vi "Result View.vi"(8 "error in (no error)":errorcluster, 11 "Coverage Report in":refnum<class "Coverage Report.lvclass">) -> (0 "error out":errorcluster, 3 "Coverage Report out":refnum<class "Coverage Report.lvclass">)   [LabVIEW 2020, in "Coverage Report.lvclass"]
uses:
  Coverage Report.lvclass
  Coverage Report.lvclass/Coverage Report.ctl
panel:
  in  "VI tree":string[](tree)
  out "Coverage Report Out":refnum<class "Coverage Report.lvclass">
  out "error out 2":errorcluster
  in  "Cancel":bool
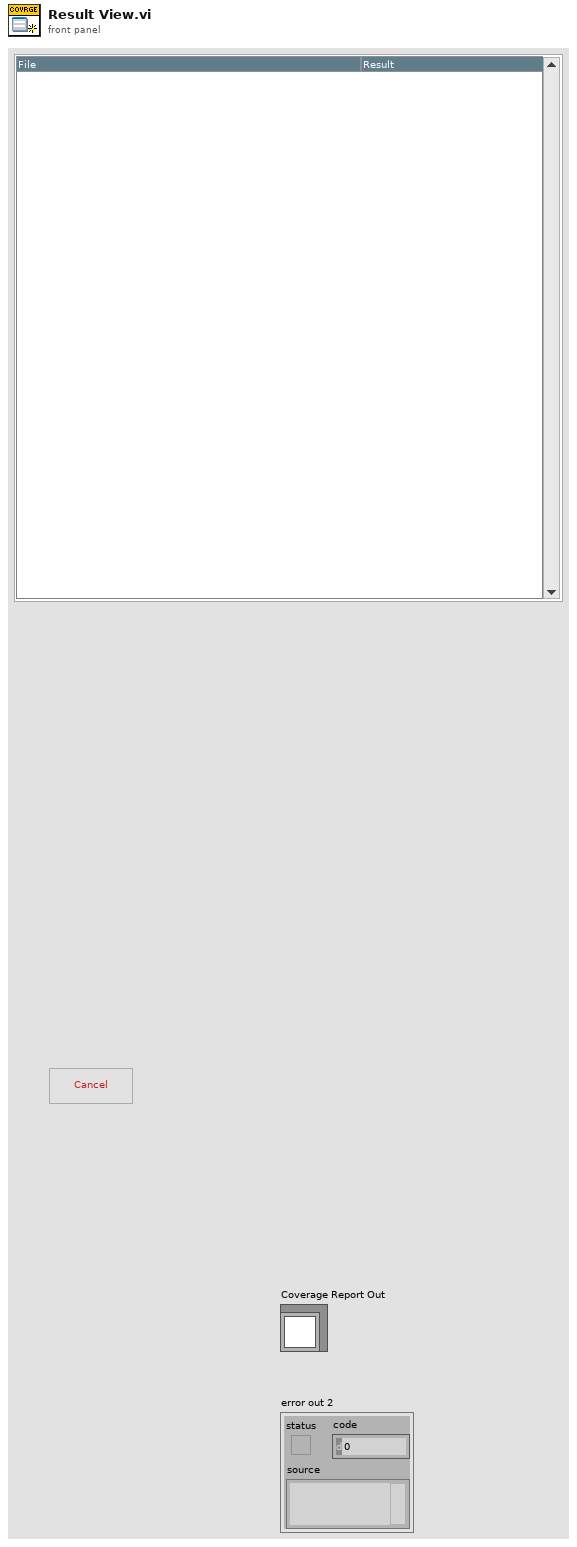
[diagram p1: front panel]
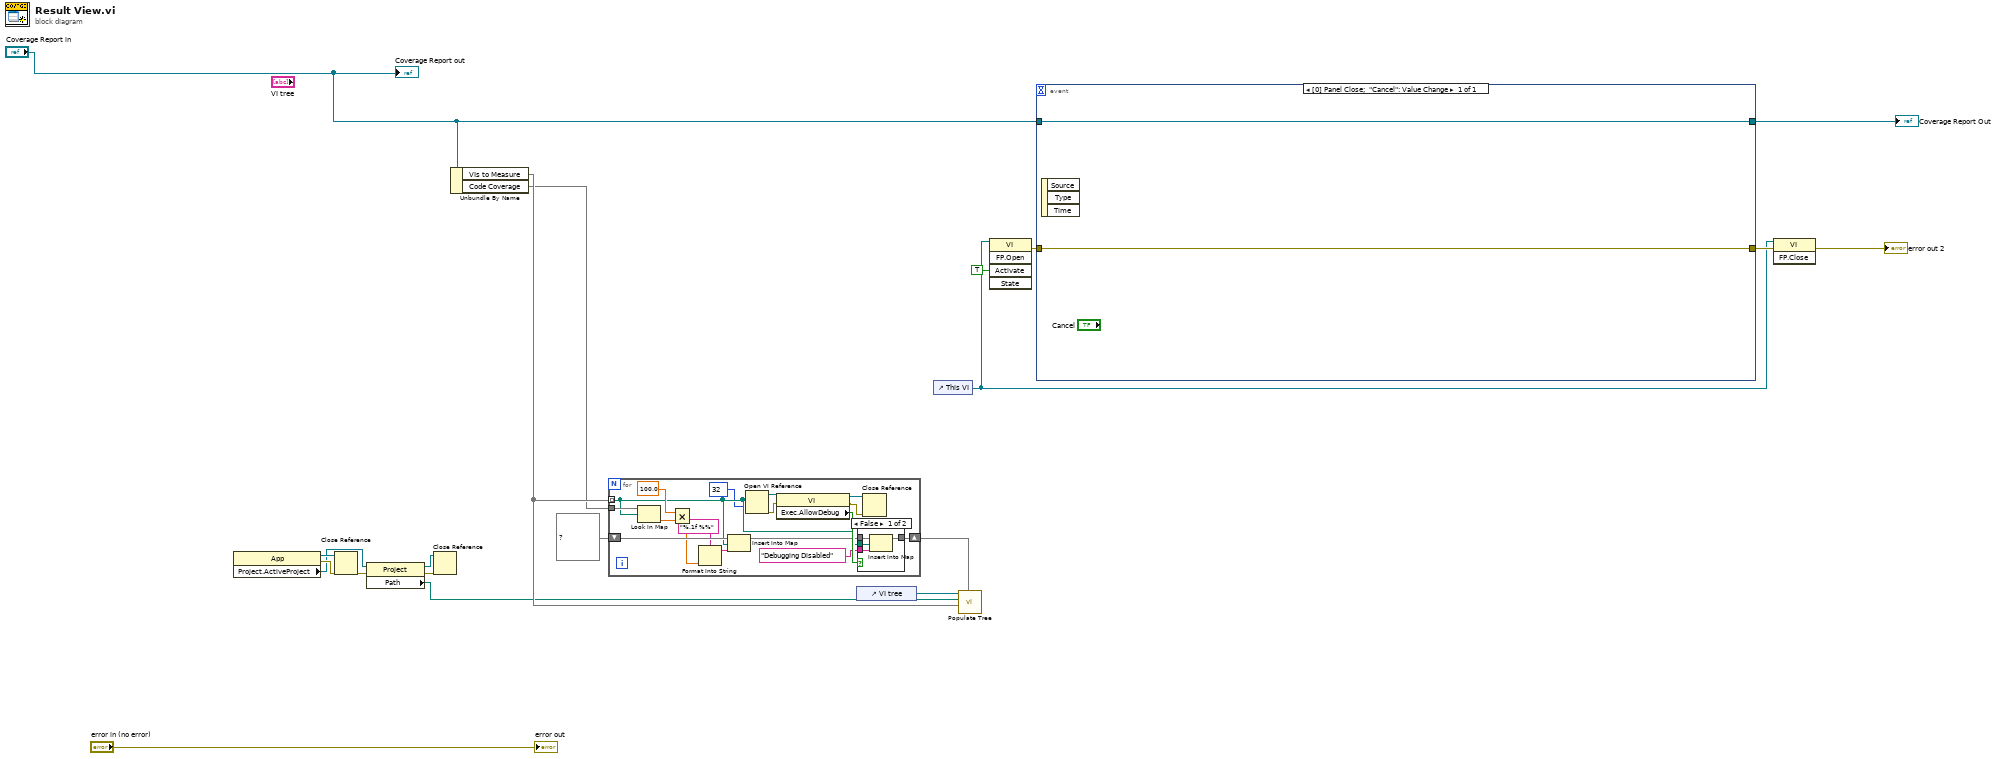
[diagram p0: block diagram]
diagram:
  n1 = property class="App"() -> (reference out=w3:refnum<vi>, error out=w6:errorcluster, "Project.ActiveProject"=w2:refnum<vi>)  [unwired: 2 in]
  n2 = Close Reference(reference=w3, error in (no error)=w6) -> (error out=w7:errorcluster)
  n3 = property class="Project"(reference=w2, error in=w7) -> (reference out=w4:refnum<vi>, error out=w5:errorcluster, "Path"=w1:path)
  n4 = Close Reference(reference=w4, error in (no error)=w5) -> ()  [unwired: 1 out]
  n5 = Unbundle By Name("Coverage Report in") -> ("VIs to Measure"=w9:set{path}, "Code Coverage"=w8:map{path, dbl})
  n6 = for {
    tunnel: w9 -> [w25] mode=indexing
    shift-right: [w32] -> w15
    shift-left: map{path, string} {} ("Results") -> [w36]
    tunnel: w8 -> [w30]
    n7 = Look In Map(map=w30, key=w25) -> (value=w28:dbl)  [unwired: 1 in, 1 out]
    n8 = Multiply(x=100.0, y=w28) -> (x*y=w23:dbl)
    n9 = Format Into String(format string="%.1f %%", w23) -> (resulting string=w26:string)  [unwired: 2 in, 1 out]
    n10 = Insert Into Map(map in=w36, key=w25, value=w26) -> (map out=w29:map{path, string})  [unwired: 2 out]
    n11 = Open VI Reference(vi path=w25, options=32) -> (vi reference=w37:refnum<vi>, error out=w34:errorcluster)  [unwired: 4 in]
    n12 = property class="VI"(reference=w37, error in=w34) -> (reference out=w35:refnum<vi>, error out=w21:errorcluster, "Exec.AllowDebug"=w33:bool)
    n13 = case shown="False" w33 {
      tunnel: w29 -> [w41 w42]
      tunnel: [w40 w42] -> w32
      tunnel: w25 -> [w39 _]
      tunnel: "Debugging Disabled" ("value") -> [w38 _]
      frame False {
        n14 = Insert Into Map(map in=w41, key=w39, value=w38) -> (map out=w40:map{path, string})  [unwired: 2 out]
      }
      frame True {
      }
    }
    n15 = Close Reference(reference=w35, error in (no error)=w21) -> ()  [unwired: 1 out]
  }
  n16 = control-ref of="VI tree"() -> (w17:refnum<vi>)
  n17 = control-ref of="This VI"() -> (w10:refnum<vi>)
  n18 = call "Populate Tree.vi"("Results"=w15, "VIs"=w9, "Project Path"=w1, "TreeControl in"=w17) -> ()  [unwired: 7 in, 1 out]
  n19 = invoke class="VI" method="FP.Open"(reference=w10, "Activate"=TRUE ("Activate?")) -> (error out=w12:errorcluster)  [unwired: 3 in, 4 out]
  n20 = event shown="[0] Panel Close;  \"Cancel\": Value Change" {
    selector: _ -> [_]
    dyn-events: _ -> [_]
    timeout: _ -> [_]
    tunnel: w12 -> [w44]
    tunnel: [w44] -> w11
    tunnel: "Coverage Report in" -> [w43]
    tunnel: [w43] -> w18
    event Panel Close; "Cancel": Value Change {
      n21 = event-data() -> ()  [unwired: 1 in, 3 out]
    }
  }
  "Coverage Report Out" <- w18
  n22 = invoke class="VI" method="FP.Close"(reference=w10, error in=w11) -> (error out=→"error out 2":errorcluster)  [unwired: 1 in, 2 out]
  "error out" <- "error in (no error)"
  "Coverage Report out" <- "Coverage Report in"
